vi "test.vi"() -> ()   [LabVIEW 2014]
panel:
  out "원소의 인덱스":i32
  out "텍스트":string[](array[string])
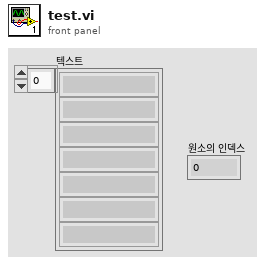
[diagram p1: front panel]
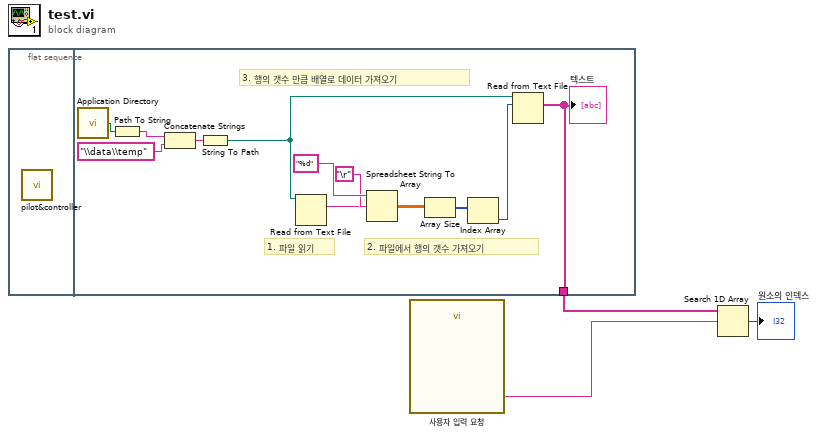
[diagram p0: block diagram]
diagram:
  n1 = flat-sequence {
    tunnel: [w4] -> w2
    frame #0 {
      n2 = call "pilot&controller.vi"() -> ()  [unwired: 11 in, 1 out]
    }
    frame #1 {
      # "3. 행의 갯수 만큼 배열로 데이터 가져오기"
      # "2. 파일에서 행의 갯수 가져오기"
      # "1. 파일 읽기"
      n3 = call <vilib>:"Application Directory.vi"() -> ("Application Directory"=w8:path)
      n4 = Path To String(path=w8) -> (string=w7:string)
      n5 = Concatenate Strings(w7, "\\data\\temp" ("문자열")) -> (w6:string)
      n6 = String To Path(string=w6) -> (path=w5:path)
      n7 = Read from Text File(file (use dialog)=w5) -> (text=w11:string)  [unwired: 1 in, 5 out]
      n8 = Spreadsheet String To Array(delimiter (Tab)="\r", format string="%d", spreadsheet string=w11) -> (array=w13:dbl[][])  [unwired: 1 out]
      n9 = Array Size(array=w13) -> (size(s)=w12:i32[])
      n10 = Index Array(array=w12) -> (element=w10:i32)  [unwired: 1 in]
      n11 = Read from Text File(file (use dialog)=w5, count=w10) -> (text=w4:string[])  [unwired: 1 in, 4 out]
      "텍스트" <- w4
    }
  }
  n12 = call "사용자 입력 요청"() -> ("nickname"=w3:string)  [unwired: 17 in, 2 out]
  n13 = Search 1D Array(1D array=w2, element=w3) -> (index of element=→"원소의 인덱스":i32)  [unwired: 1 in]
